vi "pattern_from_YAML.vi"(8 "error in (no error)":errorcluster, 11 "String":string="ncols: 2\nnrows: 2\nrotation: 0.000\nspotsize: 24.000\npitch_x: 24.000\npitch_y: 23.120\ncenter_x: 10.000\ncenter_y: -35.000\nwavelen: 5.320E-7\nsteer_lw: 1\nsteer_vmax: 95\nref_spot: 0\nfocal: 0.036\nphase_max: 3.000\nphase_factor: 82\nsteer_pad: 0\nXm: [21.72,  44.87,  68.20,  91.45, 114.72, 137.87, 160.97, 184.04]\nYm: [21.72,  44.87,  68.20,  91.45, 114.72, 137.87, 160.97, 184.04]\nphase_wrap_pos: False\nphase_wrap_neg: True\nsteer_horiz: False\ntest_pattern: False\nsteer_only: False\ngrid: True\ndark_all: False\nref_spot_dark: False\nstretch: True\n") -> (0 "error out":errorcluster, 3 "LCOS Configuration":T1 {"ref_spot" min=0 max=500 step=1 format="%#.0f"; "Y pitch" min=0.0 max=100.0 format="%.2g"; "Wavelength" min=0.0 max=500.0 format="%^#.3e"; "steer_pad" min=0 max=500 step=1 format="%#.0f"; "Steer LW" max=500; "phase_max" min=0.0 max=500.0 format="%#.3f"; "Set Focus (mm)" min=0.0 max=500.0 format="%#.3g"; "Spot size" min=1.0 format="%.2g"; "# Spots V" min=1 step=1; "# Spots H" min=1 step=1; "Center V" format="%.2f"; "Center H" format="%.2f"; "rotation" min=-90.0 max=90.0 format="%.2g"; "X pitch" min=0.0 max=100.0 format="%.2g"})   [LabVIEW 2011]
uses:
  Periodic Spot Pattern Parameters.ctl
panel:
  out "array":string[][](array[string])
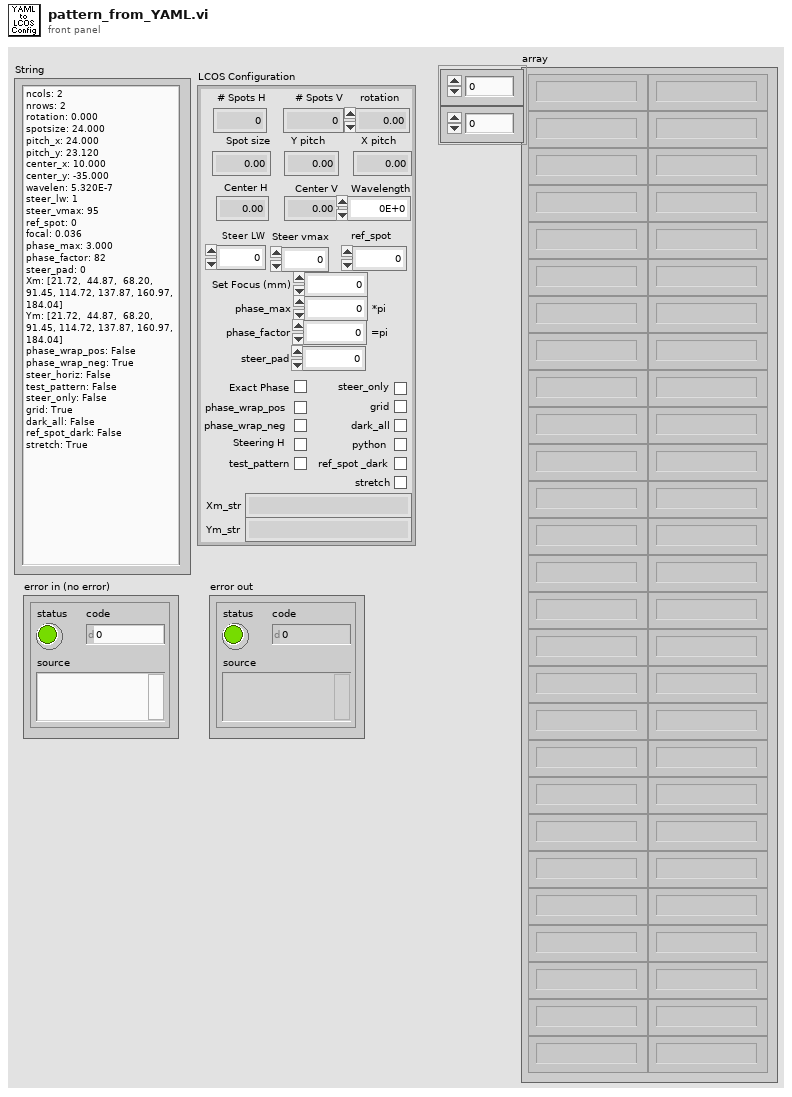
[diagram p1: front panel]
types:
  T1 = typedef "Periodic Spot Pattern Parameters.ctl" = cluster{"X pitch":dbl, "rotation":dbl, "Center H":dbl, "Center V":dbl, "# Spots H":u32, "# Spots V":u32, "Spot size":dbl, "ref_spot _dark":bool, "Exact Phase Formula":bool, "phase_wrap_pos":bool, "Set Focus (mm)":dbl, "phase_max":dbl, "phase_factor":u8, "Steer LW":u32, "Steer vmax":u8, "phase_wrap_neg":bool, "steer_horiz":bool, "steer_pad":i64, "steer_only":bool, "Wavelength":dbl, "Y pitch":dbl, "python":bool, "test_pattern":bool, "grid":bool, "dark_all":bool, "Xm_str":string, "Ym_str":string, "ref_spot":i64, "stretch":bool}
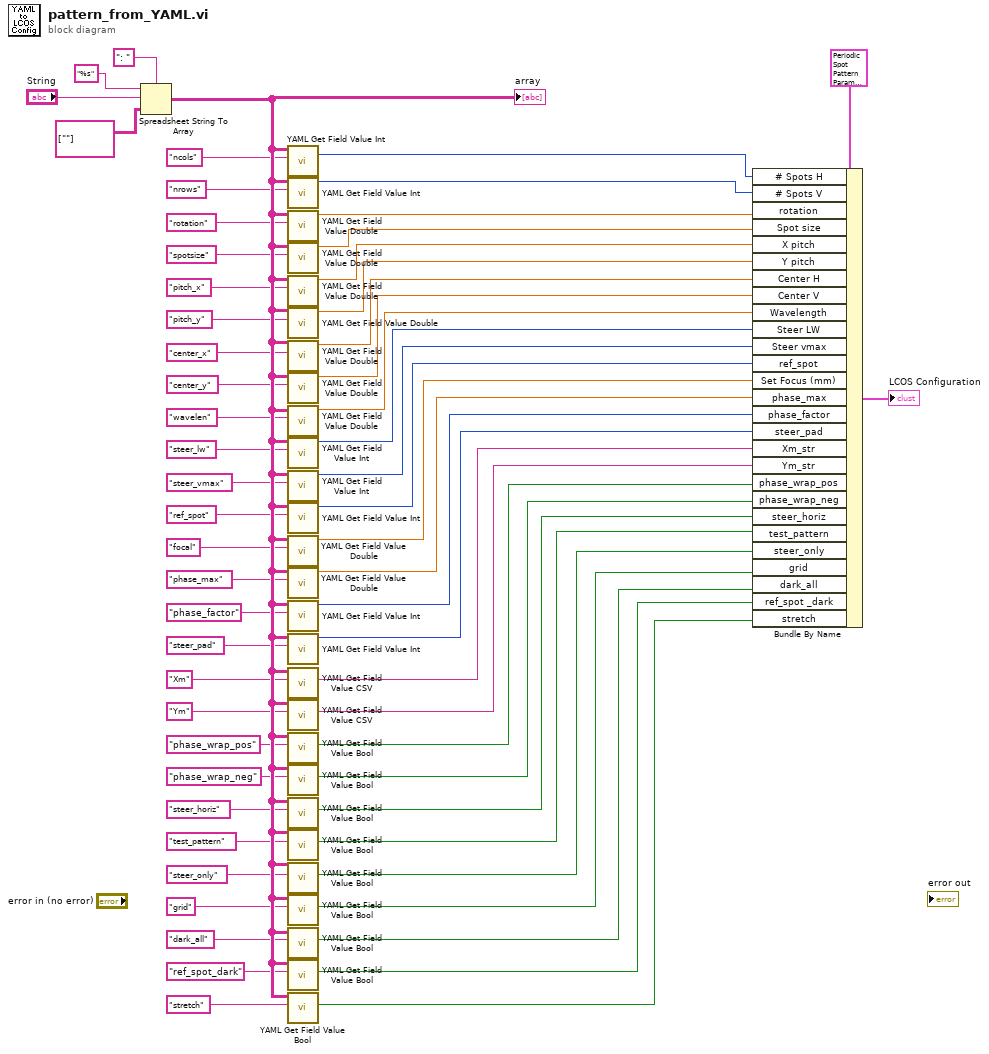
[diagram p0: block diagram]
diagram:
  n1 = Spreadsheet String To Array(delimiter (Tab)=": ", format string="%s" ("spreadsheet string"), spreadsheet string="String", array type (2D Dbl)=string[][] [[""]]) -> (array=w55:string[][])
  "array" <- w55
  n2 = call "YAML Get Field Value Int.vi"("field name"="ncols", "array of strings"=w55) -> ("Numeric Control"=w27:i32)  [unwired: 9 in]
  n3 = call "YAML Get Field Value Int.vi"("field name"="nrows", "array of strings"=w55) -> ("Numeric Control"=w26:i32)  [unwired: 9 in]
  n4 = call "YAML Get Field Value Double.vi"("field name"="rotation", "array of strings"=w55) -> ("Numeric Control"=w25:dbl)  [unwired: 9 in]
  n5 = call "YAML Get Field Value Double.vi"("field name"="spotsize", "array of strings"=w55) -> ("Numeric Control"=w24:dbl)  [unwired: 9 in]
  n6 = call "YAML Get Field Value Double.vi"("field name"="pitch_x", "array of strings"=w55) -> ("Numeric Control"=w23:dbl)  [unwired: 9 in]
  n7 = call "YAML Get Field Value Double.vi"("field name"="pitch_y", "array of strings"=w55) -> ("Numeric Control"=w22:dbl)  [unwired: 9 in]
  n8 = call "YAML Get Field Value Double.vi"("field name"="center_x", "array of strings"=w55) -> ("Numeric Control"=w21:dbl)  [unwired: 9 in]
  n9 = call "YAML Get Field Value Double.vi"("field name"="center_y", "array of strings"=w55) -> ("Numeric Control"=w20:dbl)  [unwired: 9 in]
  n10 = call "YAML Get Field Value Double.vi"("field name"="wavelen", "array of strings"=w55) -> ("Numeric Control"=w19:dbl)  [unwired: 9 in]
  n11 = call "YAML Get Field Value Int.vi"("field name"="steer_lw", "array of strings"=w55) -> ("Numeric Control"=w18:i32)  [unwired: 9 in]
  n12 = call "YAML Get Field Value Int.vi"("field name"="steer_vmax", "array of strings"=w55) -> ("Numeric Control"=w17:i32)  [unwired: 9 in]
  n13 = call "YAML Get Field Value Int.vi"("field name"="ref_spot", "array of strings"=w55) -> ("Numeric Control"=w16:i32)  [unwired: 9 in]
  n14 = call "YAML Get Field Value Double.vi"("field name"="focal", "array of strings"=w55) -> ("Numeric Control"=w15:dbl)  [unwired: 9 in]
  n15 = call "YAML Get Field Value Double.vi"("field name"="phase_max", "array of strings"=w55) -> ("Numeric Control"=w14:dbl)  [unwired: 9 in]
  n16 = call "YAML Get Field Value Int.vi"("field name"="phase_factor", "array of strings"=w55) -> ("Numeric Control"=w13:i32)  [unwired: 9 in]
  n17 = call "YAML Get Field Value Int.vi"("field name"="steer_pad", "array of strings"=w55) -> ("Numeric Control"=w12:i32)  [unwired: 9 in]
  n18 = call "YAML Get Field Value CSV.vi"("field name"="Xm", "array of strings"=w55) -> ("Field Value"=w11:string)  [unwired: 9 in]
  n19 = call "YAML Get Field Value CSV.vi"("field name"="Ym", "array of strings"=w55) -> ("Field Value"=w10:string)  [unwired: 9 in]
  n20 = call "YAML Get Field Value Bool.vi"("field name"="phase_wrap_pos", "array of strings"=w55) -> ("Boolean"=w9:bool)  [unwired: 9 in]
  n21 = call "YAML Get Field Value Bool.vi"("field name"="phase_wrap_neg", "array of strings"=w55) -> ("Boolean"=w8:bool)  [unwired: 9 in]
  n22 = call "YAML Get Field Value Bool.vi"("field name"="steer_horiz", "array of strings"=w55) -> ("Boolean"=w7:bool)  [unwired: 9 in]
  n23 = call "YAML Get Field Value Bool.vi"("field name"="test_pattern", "array of strings"=w55) -> ("Boolean"=w6:bool)  [unwired: 9 in]
  n24 = call "YAML Get Field Value Bool.vi"("field name"="steer_only", "array of strings"=w55) -> ("Boolean"=w5:bool)  [unwired: 9 in]
  n25 = call "YAML Get Field Value Bool.vi"("field name"="grid", "array of strings"=w55) -> ("Boolean"=w4:bool)  [unwired: 9 in]
  n26 = call "YAML Get Field Value Bool.vi"("field name"="dark_all", "array of strings"=w55) -> ("Boolean"=w3:bool)  [unwired: 9 in]
  n27 = call "YAML Get Field Value Bool.vi"("field name"="ref_spot_dark", "array of strings"=w55) -> ("Boolean"=w2:bool)  [unwired: 9 in]
  n28 = call "YAML Get Field Value Bool.vi"("field name"="stretch", "array of strings"=w55) -> ("Boolean"=w1:bool)  [unwired: 9 in]
  n29 = Bundle By Name(cluster=T1 {"X pitch"=0.0, "rotation"=0.0, "Center H"=0.0, "Center V"=0.0, "# Spots H"=0, "# Spots V"=0, "Spot size"=0.0, "ref_spot _dark"=FALSE, "Exact Phase Formula"=FALSE, "phase_wrap_pos"=FALSE, "Set Focus (mm)"=0.0, "phase_max"=0.0, "phase_factor"=0, "Steer LW"=0, "Steer vmax"=0, "phase_wrap_neg"=FALSE, "steer_horiz"=FALSE, "steer_pad"=0, "steer_only"=FALSE, "Wavelength"=0.0, "Y pitch"=0.0, "python"=FALSE, "test_pattern"=FALSE, "grid"=FALSE, "dark_all"=FALSE, "Xm_str"="", "Ym_str"="", "ref_spot"=0, "stretch"=FALSE} ("LCOS Configuration 2"), "# Spots H"=w27, "# Spots V"=w26, "rotation"=w25, "Spot size"=w24, "X pitch"=w23, "Y pitch"=w22, "Center H"=w21, "Center V"=w20, "Wavelength"=w19, "Steer LW"=w18, "Steer vmax"=w17, "ref_spot"=w16, "Set Focus (mm)"=w15, "phase_max"=w14, "phase_factor"=w13, "steer_pad"=w12, "Xm_str"=w11, "Ym_str"=w10, "phase_wrap_pos"=w9, "phase_wrap_neg"=w8, "steer_horiz"=w7, "test_pattern"=w6, "steer_only"=w5, "grid"=w4, "dark_all"=w3, "ref_spot _dark"=w2, "stretch"=w1) -> (→"LCOS Configuration":T1)
